vi "Get 1-Exp Global Fit Guess Parameters v2.vi"(8 "Global Fit Parameter Info":T1, 9 "IRF":cluster{"t Array":dbl[], "Data Array":dbl[]}, 11 "Full Decays":cluster{"t Array":dbl[], "Value Array":dbl[]}[](array[cluster])) -> (2 "Initial Parameters":dbl[](array[numeric])=[-1.0, 0.0, 0.5, 0.1, 0.5, 1.0])   [LabVIEW 2021, in "Fits.lvlib"]
uses:
  Global Fit Parameters Information.ctl
  Fits.lvlib
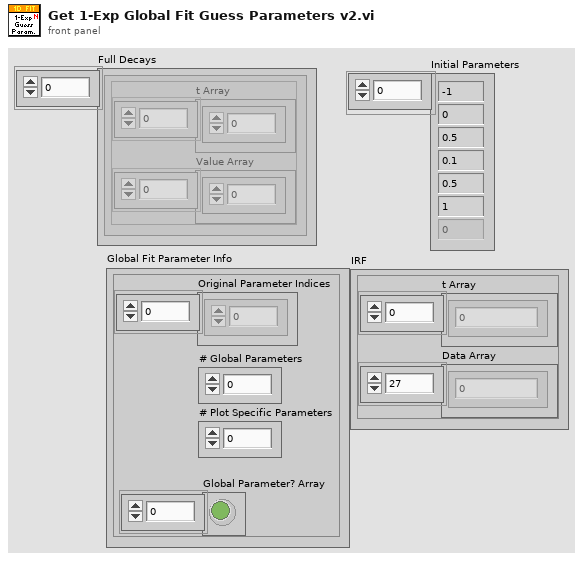
[diagram p1: front panel]
types:
  T1 = typedef "Fits.lvlib/Global Fit Parameters Information.ctl" = cluster{"Original Parameter Indices":i32[], "# Global Parameters":i32, "# Plot Specific Parameters":i32, "Global Parameter? Array":bool[]}
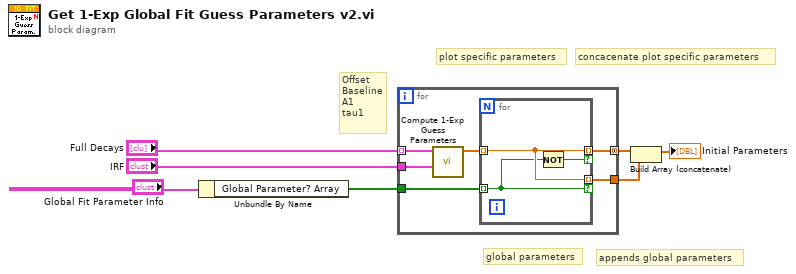
[diagram p0: block diagram]
diagram:
  # "Offset\nBaseline\nA1\ntau1"
  # "appends global parameters"
  # "concacenate plot specific parameters"
  # "plot specific parameters"
  # "global parameters"
  n1 = Unbundle By Name("Global Fit Parameter Info") -> ("Global Parameter? Array"=w5:bool[])
  n2 = for {
    tunnel: [w12] -> w7 mode=concatenating
    tunnel: w5 -> [w13]
    tunnel: [w11] -> w3
    tunnel: "Full Decays" -> [w9] mode=indexing
    tunnel: "IRF" -> [w8]
    n3 = call "Compute 1-Exp Guess Parameters.vi"("IRF"=w8, "Decay"=w9) -> ("Guess Parameters"=w10:dbl[])  [unwired: 8 in, 1 out]
    n4 = for {
      tunnel: w13 -> [w15] mode=indexing
      tunnel: w10 -> [w16] mode=indexing
      tunnel: [w16] -> w11 mode=indexing if=w15
      tunnel: [w16] -> w12 mode=indexing if=w14
      n5 = Not(x=w15) -> (.not. x?=w14:bool)
    }
  }
  n6 = Build Array (concatenate)(w7, w3) -> (→"Initial Parameters":dbl[])
